vi "Test-Control.vi"() -> ()   [LabVIEW 2014]
panel:
  out "布尔":bool caption="1231"
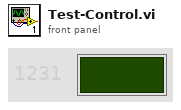
[diagram p1: front panel]
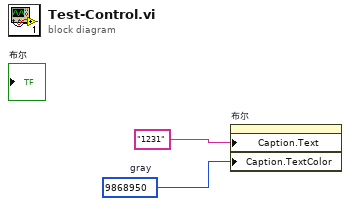
[diagram p0: block diagram]
diagram:
  w1 = u32 9868950  # gray
  n1 = property on="布尔" class="Bool (严格)"("Caption.Text"="1231" ("标题.文本"), "Caption.TextColor"=w1) -> ()  [unwired: 2 in, 2 out]
